vi "Multi (Selector).vi"(8 "error in (no error)":errorcluster, 9 "Constant":dbl=1.0, 10 "Aux Data Sources":T1) -> (0 "error out":errorcluster, 3 "Multi out":refnum<class "Multi.lvclass">)   [LabVIEW 2009, in "Multi.lvclass"]
uses:
  Multi.lvclass
  Aux Data Source/Aux Data Source.lvclass
  Norm/Norm.lvclass
  Normalize/Normalize.lvclass
  Polarization/Polarization.lvclass
  Plus/Plus.lvclass
  Difference/Difference.lvclass
  Average/Average.lvclass
  Multiply/Multiply.lvclass
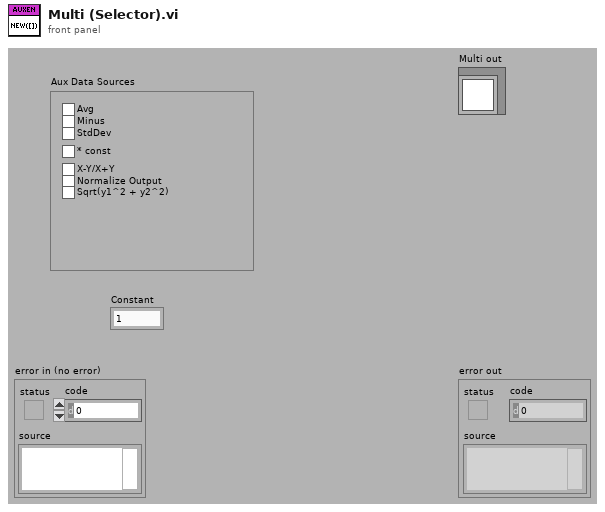
[diagram p1: front panel]
types:
  T1 = cluster{"Avg":bool, "Minus":bool, "StdDev":bool, "* const":bool, "X-Y/X+Y":bool, "Normalize Output":bool, "Sqrt(y1^2 + y2^2)":bool}
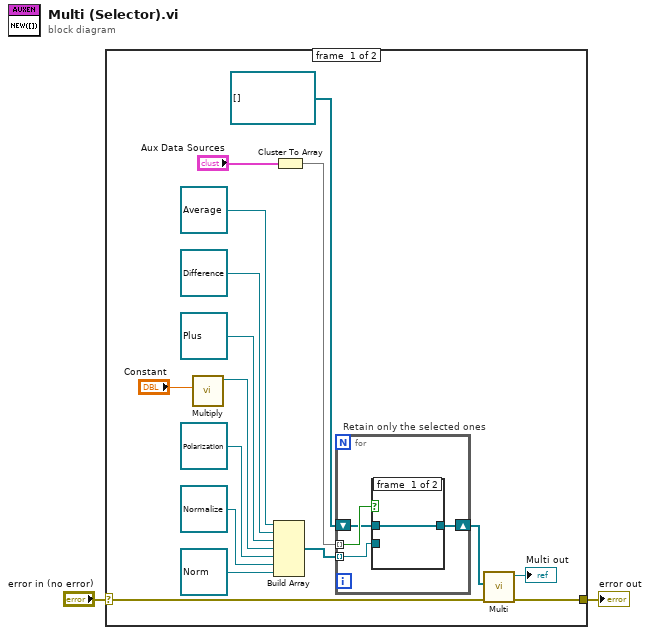
[diagram p0: block diagram]
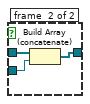
[diagram p2: hidden frame]
diagram:
  n1 = case shown="No Error" "error in (no error)" {
    selector: "error in (no error)" -> [w8 w27]
    tunnel: [w7 w27] -> w1
    frame #0 {
      n2 = call "Multiply.vi"("Constant"="Constant") -> ("Multiply out"=w14:refnum<class "Multiply.lvclass">)  [unwired: 9 in, 1 out]
      n3 = Build Array(refnum<class "Average.lvclass"> refnum ("Average.lvclass"), refnum<class "Difference.lvclass"> refnum ("Difference.lvclass"), refnum<class "Plus.lvclass"> refnum ("Plus.lvclass"), w14, refnum<class "Polarization.lvclass"> refnum ("Polarization.lvclass"), refnum<class "Normalize.lvclass"> refnum ("Normalize.lvclass"), refnum<class "Norm.lvclass"> refnum ("Norm.lvclass")) -> (w10:refnum<class "Aux Data Source.lvclass">[])
      n4 = Cluster To Array(cluster="Aux Data Sources") -> (array=w11:bool[])
      n5 = for "Retain only the selected ones" {
        tunnel: w11 -> [w21] mode=indexing
        tunnel: w10 -> [w22] mode=indexing
        shift-right: [w19] -> w9
        shift-left: refnum<class "Aux Data Source.lvclass">[] [] -> [w20]
        n6 = case shown="True" w21 {
          tunnel: w22 -> [_ w25]
          tunnel: [w23 w26] -> w19
          tunnel: w20 -> [w23 w24]
          frame #0 {
          }
          frame #1 {
            n7 = Build Array (concatenate)(w24, w25) -> (w26:refnum<class "Aux Data Source.lvclass">[])
          }
        }
      }
      n8 = call "Multi.vi"("error in (no error)"=w8, "Data Sources"=w9) -> ("error out"=w7:errorcluster, "Multi out"=→"Multi out":refnum<class "Multi.lvclass">)  [unwired: 8 in]
    }
    frame #1 {
    }
  }
  "error out" <- w1
